vi "Handle getAll.vi"(8 "error in (no error)":errorcluster, 11 "instrument.PPMS in":refnum<class "instrument.PPMS.lvclass">) -> (0 "error out":errorcluster, 2 "getAll":variant, 3 "instrument.PPMS out":refnum<class "instrument.PPMS.lvclass">)   [LabVIEW 2019, in "instrument.PPMS.lvclass"]
uses:
  instrument.PPMS.lvclass
  Typedefs/PPMS.getAll--cluster.ctl
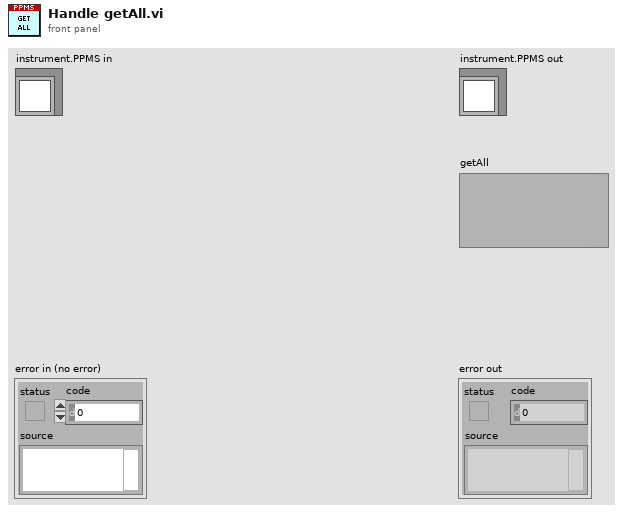
[diagram p1: front panel]
types:
  T1 = typedef "instrument.PPMS.lvclass/PPMS.getAll--cluster.ctl" = cluster{"Chamber Status":string, "Helium Level (%)":dbl, "Temperature (K)":dbl, "Temperature Status":string, "Magnetic Field (T)":dbl, "Magnet Status":string, "Position (°)":dbl}
  T2 = typedef "instrument.PPMS.lvclass/PPMS.Temperature Status--cluster.ctl" = cluster{"Temperature (K)":dbl, "Temperature Status":string}
  T3 = typedef "instrument.PPMS.lvclass/PPMS.Magnet Status--cluster.ctl" = cluster{"Field (T)":dbl, "Magnet Status":string}
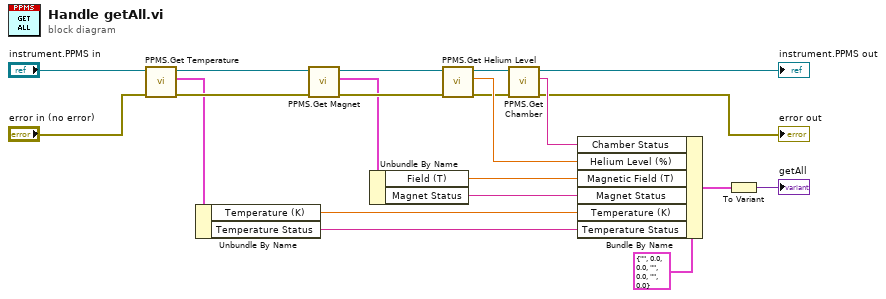
[diagram p0: block diagram]
diagram:
  n1 = call "PPMS.Get Temperature.vi"("error in (no error)"="error in (no error)", "instrument.PPMS"="instrument.PPMS in") -> ("error out"=w18:errorcluster, "Temperature Status"=w7:T2, "instrument.PPMS out"=w20:refnum<class "instrument.PPMS.lvclass">)  [unwired: 7 in]
  n2 = Unbundle By Name(w7) -> ("Temperature (K)"=w16:dbl, "Temperature Status"=w15:string)
  n3 = call "PPMS.Get Magnet.vi"("error in (no error)"=w18, "instrument.PPMS"=w20) -> ("error out"=w17:errorcluster, "Magnet Status"=w6:T3, "instrument.PPMS out"=w19:refnum<class "instrument.PPMS.lvclass">)  [unwired: 7 in]
  n4 = Unbundle By Name(w6) -> ("Field (T)"=w13:dbl, "Magnet Status"=w14:string)
  n5 = call "PPMS.Get Helium Level.vi"("error in (no error)"=w17, "instrument.PPMS"=w19) -> ("error out"=w4:errorcluster, "Helium Level (%)"=w12:dbl, "instrument.PPMS out"=w5:refnum<class "instrument.PPMS.lvclass">)  [unwired: 7 in]
  n6 = call "PPMS.Get Chamber.vi"("error in (no error)"=w4, "instrument.PPMS"=w5) -> ("error out"=→"error out":errorcluster, "Status String"=w2:string, "instrument.PPMS out"=→"instrument.PPMS out":refnum<class "instrument.PPMS.lvclass">)  [unwired: 7 in]
  n7 = Bundle By Name(cluster=T1 {"Chamber Status"="", "Helium Level (%)"=0.0, "Temperature (K)"=0.0, "Temperature Status"="", "Magnetic Field (T)"=0.0, "Magnet Status"="", "Position (°)"=0.0} ("getAll"), "Chamber Status"=w2, "Helium Level (%)"=w12, "Magnetic Field (T)"=w13, "Magnet Status"=w14, "Temperature (K)"=w16, "Temperature Status"=w15) -> (w21:T1)
  n8 = To Variant(anything=w21) -> (Variant=→"getAll":variant)
